vi "PhotonTrackedTarget_Equals.vi"(9 "Other TrackedTarget":T1={"Yaw"=0.0, "Pitch"=0.0, "Area"=0.0, "Skew"=0.0, "MinAreaRectCorners"=[], "BestCameraToTarget"={"TRANSLATION3D"={"X"=0.0, "Y"=0.0, "Z"=0.0}, "ROTATION3D"={"Q_quaternion"={"R"=1.0, "V"=[0.0, 0.0, 0.0]}}, "XF"=FALSE}, "FiiducialId"=0, "AltCameraToTarget"={"TRANSLATION3D"={"X"=0.0, "Y"=0.0, "Z"=0.0}, "ROTATION3D"={"Q_quaternion"={"R"=1.0, "V"=[0.0, 0.0, 0.0]}}, "XF"=FALSE}, "PoseAmbiguity"=0.0, "DetectedCorners"=[]} {"AltCameraToTarget"."TRANSLATION3D"."Z" format="%14.3f"; "AltCameraToTarget"."TRANSLATION3D"."Y" format="%14.3f"; "AltCameraToTarget"."TRANSLATION3D"."X" format="%14.3f"; "BestCameraToTarget"."TRANSLATION3D"."Z" format="%14.3f"; "BestCameraToTarget"."TRANSLATION3D"."Y" format="%14.3f"; "BestCameraToTarget"."TRANSLATION3D"."X" format="%14.3f"}, 11 "TrackedTarget":T1={"Yaw"=0.0, "Pitch"=0.0, "Area"=0.0, "Skew"=0.0, "MinAreaRectCorners"=[], "BestCameraToTarget"={"TRANSLATION3D"={"X"=0.0, "Y"=0.0, "Z"=0.0}, "ROTATION3D"={"Q_quaternion"={"R"=1.0, "V"=[0.0, 0.0, 0.0]}}, "XF"=FALSE}, "FiiducialId"=0, "AltCameraToTarget"={"TRANSLATION3D"={"X"=0.0, "Y"=0.0, "Z"=0.0}, "ROTATION3D"={"Q_quaternion"={"R"=1.0, "V"=[0.0, 0.0, 0.0]}}, "XF"=FALSE}, "PoseAmbiguity"=0.0, "DetectedCorners"=[]} {"AltCameraToTarget"."TRANSLATION3D"."Z" format="%14.3f"; "AltCameraToTarget"."TRANSLATION3D"."Y" format="%14.3f"; "AltCameraToTarget"."TRANSLATION3D"."X" format="%14.3f"; "BestCameraToTarget"."TRANSLATION3D"."Z" format="%14.3f"; "BestCameraToTarget"."TRANSLATION3D"."Y" format="%14.3f"; "BestCameraToTarget"."TRANSLATION3D"."X" format="%14.3f"}) -> (3 "Equals":bool)   [LabVIEW 2019, in "PhotonVisionLib.lvlib"]
doc: "Determines if two tracked targets are equal\n\nInputs:\n - TrackedTarget -- TrackedTarget cluster.\n - OtherTrackedTarget -- Second TrackedTarget cluster.\n\nOutputs:\n - Area -- Boolean, equals TRUE if both TrackedTargets are the same."
uses:
  PhotonVisionLib.lvlib
  TypeDef/PhotonTrackedTargetType.ctl
  TypeDef/TargetCornerType.ctl
  <vilib>/Rock Robotics/WPI/ThirdParty/JAS_Junk/TrajLib/TypeDef/TRANSFORM3D.ctl
  <vilib>/Rock Robotics/WPI/ThirdParty/JAS_Junk/TrajLib/TypeDef/TRANSLATION3D.ctl
  <vilib>/Rock Robotics/WPI/ThirdParty/JAS_Junk/TrajLib/TypeDef/ROTATION3D.ctl
  <vilib>/Rock Robotics/WPI/ThirdParty/JAS_Junk/TrajLib/TypeDef/QUATERNION.ctl
  <vilib>/Rock Robotics/WPI/ThirdParty/JAS_Junk/TrajLib/VI/Transform3d_GetTranslation3d.vi
  <vilib>/Rock Robotics/WPI/ThirdParty/JAS_Junk/TrajLib/VI/Transform3d_GetRotation3d.vi
  <vilib>/Rock Robotics/WPI/ThirdParty/JAS_Junk/TrajLib/VI/Rotation3d_Equals.vi
  <vilib>/Rock Robotics/WPI/ThirdParty/JAS_Junk/TrajLib/VI/Translation3d_Equals.vi
  <vilib>/Rock Robotics/WPI/ThirdParty/JAS_Junk/TrajLib/VI/Rotation3d_GetQuaterion.vi
  <vilib>/Rock Robotics/WPI/ThirdParty/JAS_Junk/TrajLib/VI/Quaternion_Equals.vi
  <vilib>/Rock Robotics/WPI/ThirdParty/JAS_Junk/TrajLib/VI/Quaternion_Get_Vect.vi
  <vilib>/Rock Robotics/WPI/ThirdParty/JAS_Junk/TrajLib/VI/Quaternion_Get_W.vi
  <vilib>/Rock Robotics/WPI/ThirdParty/JAS_Junk/TrajLib/Trajectory_Library.lvlib
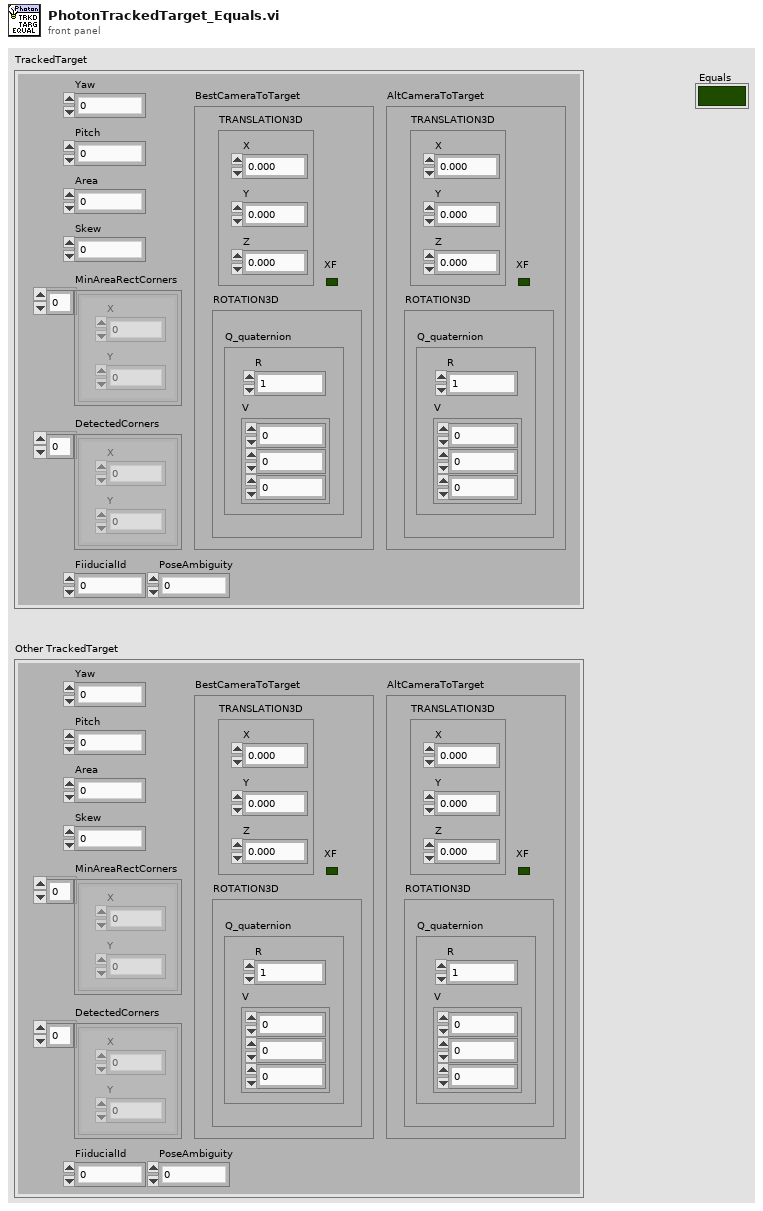
[diagram p1: front panel]
types:
  T1 = typedef "PhotonVisionLib.lvlib/PhotonTrackedTargetType.ctl" = cluster{"Yaw":dbl, "Pitch":dbl, "Area":dbl, "Skew":dbl, "MinAreaRectCorners":T2[], "BestCameraToTarget":T3, "FiiducialId":i32, "AltCameraToTarget":T3, "PoseAmbiguity":dbl, "DetectedCorners":T2[]}
  T2 = typedef "PhotonVisionLib.lvlib/TargetCornerType.ctl" = cluster{"X":dbl, "Y":dbl}
  T3 = typedef "Trajectory_Library.lvlib/TRANSFORM3D.ctl" = cluster{"TRANSLATION3D":T4, "ROTATION3D":T5, "XF":bool}
  T4 = typedef "Trajectory_Library.lvlib/TRANSLATION3D.ctl" = cluster{"X":dbl, "Y":dbl, "Z":dbl}
  T5 = typedef "Trajectory_Library.lvlib/ROTATION3D.ctl" = cluster{"Q_quaternion":T6}
  T6 = typedef "Trajectory_Library.lvlib/QUATERNION.ctl" = cluster{"R":dbl, "V":dbl[]}
  T7 = cluster{"Yaw":bool, "Pitch":bool, "Area":bool, "Skew":bool, "MinAreaRectCorners":cluster{"X":bool, "Y":bool}[], "BestCameraToTarget":cluster{"TRANSLATION3D":cluster{"X":bool, "Y":bool, "Z":bool}, "ROTATION3D":cluster{"Q_quaternion":cluster{"R":bool, "V":bool[]}}, "XF":bool}, "FiiducialId":bool, "AltCameraToTarget":cluster{"TRANSLATION3D":cluster{"X":bool, "Y":bool, "Z":bool}, "ROTATION3D":cluster{"Q_quaternion":cluster{"R":bool, "V":bool[]}}, "XF":bool}, "PoseAmbiguity":bool, "DetectedCorners":cluster{"X":bool, "Y":bool}[]}
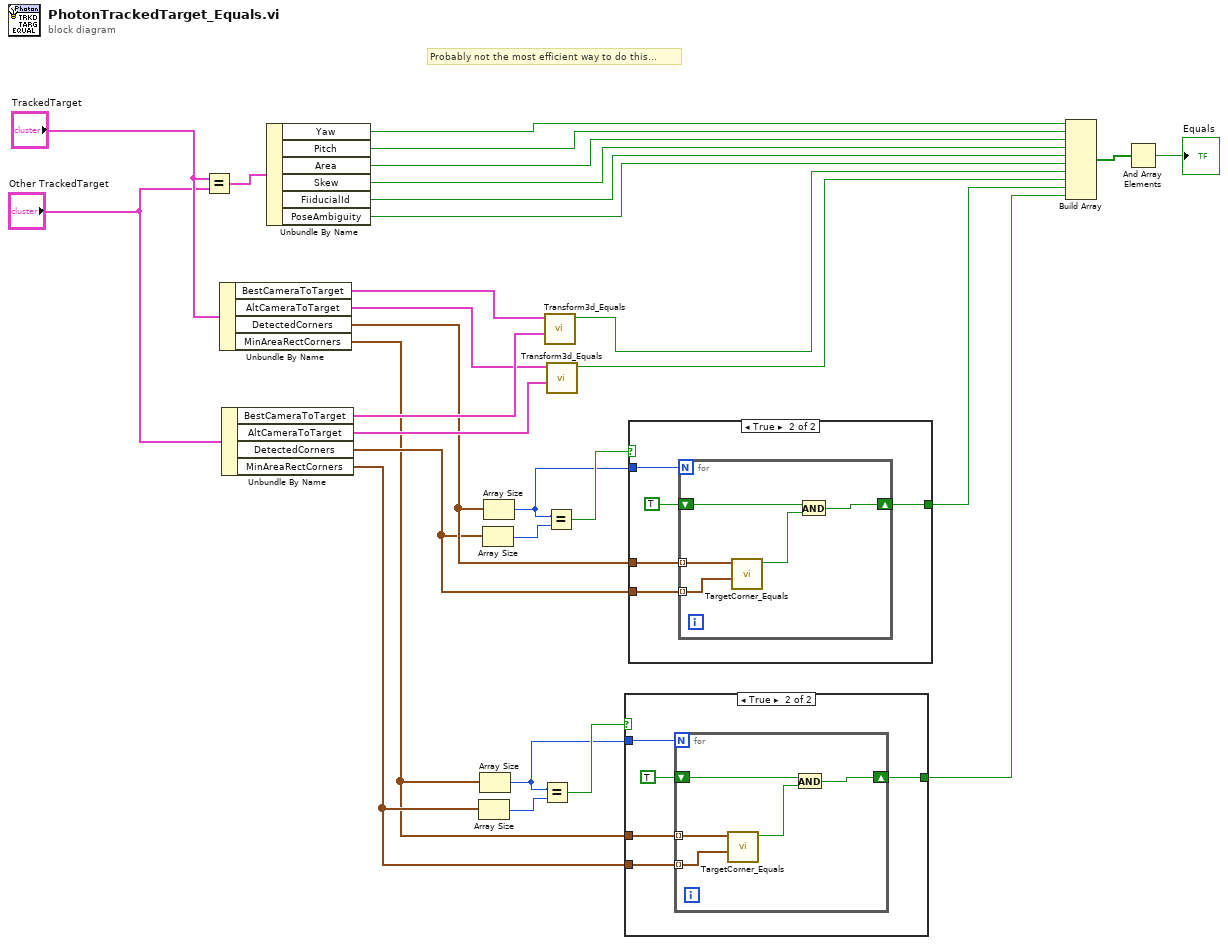
[diagram p0: block diagram]
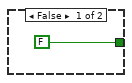
[diagram p2: hidden frame]
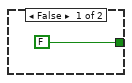
[diagram p3: hidden frame]
diagram:
  # "Probably not the most efficient way to do this..."
  n1 = Equal?(x="TrackedTarget", y="Other TrackedTarget") -> (x = y?=w29:T7)
  n2 = Unbundle By Name("TrackedTarget") -> ("BestCameraToTarget"=w18:T3, "AltCameraToTarget"=w16:T3, "DetectedCorners"=w9:T2[], "MinAreaRectCorners"=w2:T2[])
  n3 = Unbundle By Name("Other TrackedTarget") -> ("BestCameraToTarget"=w17:T3, "AltCameraToTarget"=w15:T3, "DetectedCorners"=w8:T2[], "MinAreaRectCorners"=w3:T2[])
  n4 = Unbundle By Name(w29) -> ("Yaw"=w28:bool, "Pitch"=w27:bool, "Area"=w26:bool, "Skew"=w25:bool, "FiiducialId"=w24:bool, "PoseAmbiguity"=w23:bool)
  n5 = Array Size(array=w3) -> (size(s)=w6:i32)
  n6 = Array Size(array=w2) -> (size(s)=w4:i32)
  n7 = Array Size(array=w8) -> (size(s)=w12:i32)
  n8 = Array Size(array=w9) -> (size(s)=w10:i32)
  n9 = Equal?(x=w4, y=w6) -> (x = y?=w5:bool)
  n10 = call <vilib>:"Transform3d_Equals.vi"("otherTransform3d"=w17, "inTransform3d"=w18) -> ("Equals"=w14:bool)  [unwired: 9 in]
  n11 = Equal?(x=w10, y=w12) -> (x = y?=w11:bool)
  n12 = call <vilib>:"Transform3d_Equals.vi"("otherTransform3d"=w15, "inTransform3d"=w16) -> ("Equals"=w13:bool)  [unwired: 9 in]
  n13 = case shown="True" w5 {
    tunnel: [FALSE w31] -> w1
    tunnel: w4 -> [_ w34]
    tunnel: w2 -> [_ w33]
    tunnel: w3 -> [_ w32]
    frame False {
    }
    frame True {
      n14 = for {
        N: w34 -> [_]
        shift-right: [w39] -> w31
        shift-left: TRUE -> [w40]
        tunnel: w33 -> [w38] mode=indexing
        tunnel: w32 -> [w37] mode=indexing
        n15 = call "TargetCorner_Equals.vi"("Other TargetCorner"=w37, "TargetCorner"=w38) -> ("Equals"=w36:bool)  [unwired: 9 in]
        n16 = And(x=w40, y=w36) -> (x .and. y?=w39:bool)
      }
    }
  }
  n17 = case shown="True" w11 {
    tunnel: [FALSE w42] -> w7
    tunnel: w10 -> [_ w45]
    tunnel: w9 -> [_ w44]
    tunnel: w8 -> [_ w43]
    frame False {
    }
    frame True {
      n18 = for {
        N: w45 -> [_]
        shift-right: [w50] -> w42
        shift-left: TRUE -> [w51]
        tunnel: w44 -> [w49] mode=indexing
        tunnel: w43 -> [w48] mode=indexing
        n19 = call "TargetCorner_Equals.vi"("Other TargetCorner"=w48, "TargetCorner"=w49) -> ("Equals"=w47:bool)  [unwired: 9 in]
        n20 = And(x=w51, y=w47) -> (x .and. y?=w50:bool)
      }
    }
  }
  n21 = Build Array(w28, w27, w26, w25, w24, w23, w14, w13, w7, w1) -> (w22:bool[])
  n22 = And Array Elements(Boolean array=w22) -> (logical AND=→"Equals":bool)
